vi "Practica 3.vi"() -> ()   [LabVIEW 2018]
uses:
  <vilib>/LabVIEW Interface for Arduino/Type Defs/Digital Pin.ctl
  <vilib>/LabVIEW Interface for Arduino/Type Defs/Pin Mode.ctl
  <vilib>/LabVIEW Interface for Arduino/LabVIEW Interface for Arduino.lvlib
panel:
  out "Array":bool[](array[boolean])
  in  "stop":bool
  in  "PIN Digital":T1
  # "Practica 3: Entrada Digital"
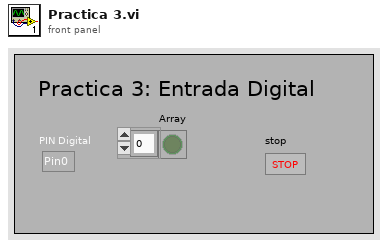
[diagram p1: front panel]
types:
  T1 = typedef "LabVIEW Interface for Arduino.lvlib/Digital Pin.ctl" = enum8{"Pin0", "Pin1", "Pin2", "Pin3", "Pin4", "Pin5", "Pin6", "Pin7", "Pin8", "Pin9", "Pin10", "Pin11", "Pin12", "Pin13"}
  T2 = typedef "LabVIEW Interface for Arduino.lvlib/Arduino Resource.ctl" = cluster{"VISA resource":refnum<visa-resource-name>, "Board Type":T3, "Connection Type":enum8{"USB / Serial"}, "Bytes Per Packet (15)":u8}
  T3 = typedef "LabVIEW Interface for Arduino.lvlib/Board Type.ctl" = enum16{"Uno", "Dimuelanove w/Atmega 328", "Mega 2560"}
  T4 = typedef "LabVIEW Interface for Arduino.lvlib/Pin Mode.ctl" = enum8{"Input", "Output"}
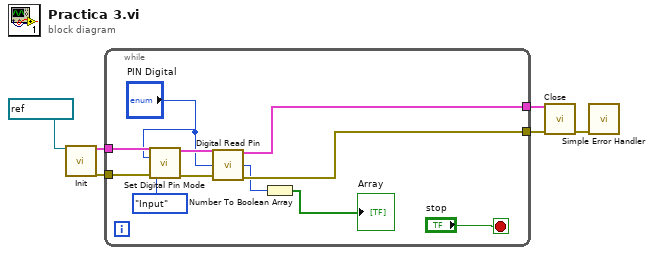
[diagram p0: block diagram]
diagram:
  n1 = call <vilib>:"Init.vi"("VISA resource"=refnum<visa-resource-name> "COM9") -> ("Arduino Resource"=w4:T2, "error out"=w3:errorcluster)  [unwired: 17 in]
  n2 = while {
    tunnel: w4 -> [w16]
    tunnel: w3 -> [w15]
    tunnel: [w10] -> w2
    tunnel: [w9] -> w1
    stop <- "stop" stop-if-true
    n3 = call <vilib>:"Set Digital Pin Mode.vi"("Arduino Resource"=w16, "Digital I/O Pin"="PIN Digital", "Pin Mode (Input)"=Pin_Mode."Input", "error in"=w15) -> ("Arduino Resource"=w14:T2, "error out"=w13:errorcluster)  [unwired: 10 in]
    n4 = call <vilib>:"Digital Read Pin.vi"("Arduino Resource"=w14, "Digital I/O Pin (0)"="PIN Digital", "error in"=w13) -> ("Arduino Resource"=w10:T2, "Value"=w8:u8, "error out"=w9:errorcluster)  [unwired: 10 in]
    n5 = Number To Boolean Array(number=w8) -> (Boolean array=→"Array":bool[])
  }
  n6 = call <vilib>:"Close.vi"("Arduino Resource"=w2, "error in"=w1) -> ("error out"=w5:errorcluster)  [unwired: 13 in]
  n7 = call <vilib>:"Simple Error Handler.vi"("error in (no error)"=w5) -> ()  [unwired: 4 in, 5 out]
